vi "GenNet Close UDP Connection.vi"(8 "error in (no error)":errorcluster, 11 "UDP Network Connection in":refnum<k16>) -> (0 "error out":errorcluster, 3 "UDP Network Connection out":refnum<k16>)   [LabVIEW 2022 SP3, in "hse-gennet.lvlib"]
doc: "Closes a TCP/IP connection.\n\n____\nHAMPEL SOFTWARE ENGINEERING v3.8.0 (2023-12-18 14:41)"
uses:
  hse-gennet.lvlib
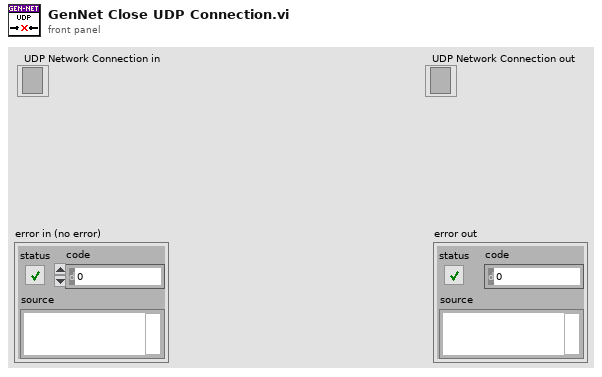
[diagram p1: front panel]
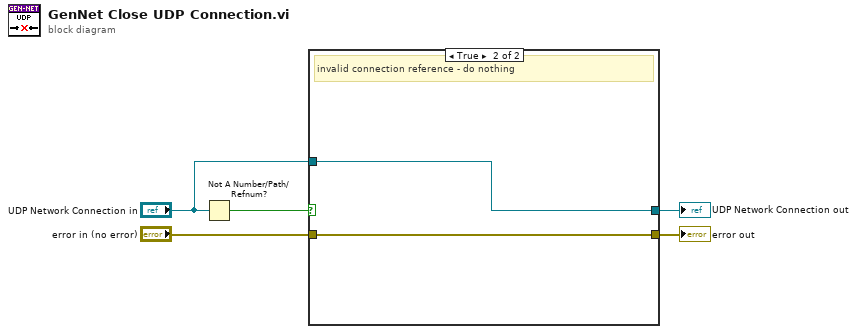
[diagram p0: block diagram]
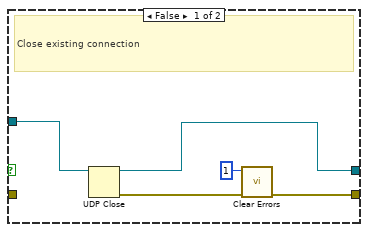
[diagram p2: hidden frame]
diagram:
  n1 = Not A Number/Path/Refnum?(number/path/refnum="UDP Network Connection in") -> (NaN/Path/Refnum?=w3:bool)
  n2 = case shown="True" w3 {
    tunnel: [w7 w11] -> w2
    tunnel: [w10 w12] -> w5
    tunnel: "error in (no error)" -> [_ w12]
    tunnel: "UDP Network Connection in" -> [w8 w11]
    frame False {
      # "Close existing connection"
      n3 = UDP Close(connection ID=w8) -> (connection ID out=w7:refnum<k16>, error out=w6:errorcluster)  [unwired: 1 in]
      n4 = call <vilib>:"Clear Errors.vi"("error in (no error)"=w6, "specific error code to clear (0: all)"=1) -> ("error out"=w10:errorcluster)  [unwired: 4 in, 1 out]
    }
    frame True {
      # "invalid connection reference - do nothing"
    }
  }
  "error out" <- w5
  "UDP Network Connection out" <- w2
